vi "setting page.vi"(5 "NAN error":i32, 11 "error constant":errorcluster) -> (3 "sensor cluster":T5={"ch sensor1"=2.0, "ch sensor2"=3.0, "chs ensor3"=4.0, "ch sw sensor1"=0.0, "ch sw sensor2"=1.0}, 4 "This VI":refnum<vi>, 6 "grtbar":T3={"level1 thr"=5.0, "level2 thr"=10.0, "gr.th1"=900.0, "gr.th2"=900.0, "gr.th3"=900.0, "gr.th4"=900.0, "gr.th5"=18000.0, "gr.th6"=20000.0, "gr.th7"=21000.0, "gr.th8"=22000.0, "gr.th9"=3000.0, "def size"=5.0, "Frame False Thr"=280.0}, 8 "curv cluster":T2={"Thr1"=40000.0, "Thr2"=40000.0, "Thr3"=40000.0, "Port"=502.0, "time out"=50.0, "SWR thr"=20000.0, "SWL thr "=20000.0, "Curv thr (mm)"=13.0, "SW timout(s)"=0.25, "falling level thr"=59000.0, "denoise thr1"=20000.0, "denoise thr2"=20000.0, "denoise thr3"=20000.0, "low level read thr"=39000.0, "Debounce Time"=0.5}, 10 "IP # 2":string="169.254.116.245", 13 "general setting":T1={"plt number dis"=45, "Table Name"="pallet", "Database Name"="PALLETCAR", "DB days to save"=3}, 14 "counting role":T4(ring), 15 "img path 2":path=path "C:/Users/user/Pictures/saved pic")   [LabVIEW 2019]
panel:
  out "NAN Error":i32
  out "error constant 2":errorcluster
  out "Errors":string
  in  "DB days to save":i16=3
  in  "Debounce Time":dbl=0.5
  in  "counting role 2":T4(ring) caption="counting role"
  in  "Frame False Thr":dbl=280.0
  in  "ch sw sensor1":dbl
  out "Side Wall Setting":string
  in  "Port":dbl=502.0
  in  "SWL thr":dbl=20000.0
  in  "denoise thr3":dbl=20000.0
  in  "denoise thr2":dbl=20000.0
  in  "low level read thr":dbl=39000.0
  in  "denoise thr1":dbl=20000.0
  in  "falling level thr":dbl=59000.0
  in  "Database Name":string="PALLETCAR"
  in  "plt number dis":i16=45
  in  "Table Name":string="pallet"
  out "General Setting":string
  in  "SW timout(s)":dbl=0.25
  in  "Curv thr (mm)":dbl=13.0
  in  "SWR thr":dbl=20000.0
  in  "ch sw sensor2":dbl=1.0
  in  "chs ensor3":dbl=4.0
  in  "ch sensor2":dbl=3.0
  in  "ch sensor1":dbl=2.0
  in  "gr.th7":dbl=21000.0
  in  "gr.th8":dbl=22000.0
  in  "gr.th9":dbl=3000.0
  in  "Thr3":dbl=40000.0
  out "Gratebar Setting":string
  in  "gr.th6":dbl=20000.0
  in  "gr.th5":dbl=18000.0
  in  "gr.th4":dbl=900.0
  in  "gr.th3":dbl=900.0
  in  "gr.th2":dbl=870.0
  in  "gr.th1":dbl=850.0
  in  "IP #":string="169.254.116.245"
  out "Curve Setting":string
  in  "def size":dbl=5.0
  in  "Img Path":path=path "C:/Users/user/Pictures/saved pic"
  in  "level2 thr":dbl=50.0
  in  "level1 thr":dbl=25.0
  in  "time out":dbl=50.0
  in  "Thr2":dbl=40000.0
  in  "Thr1":dbl=40000.0
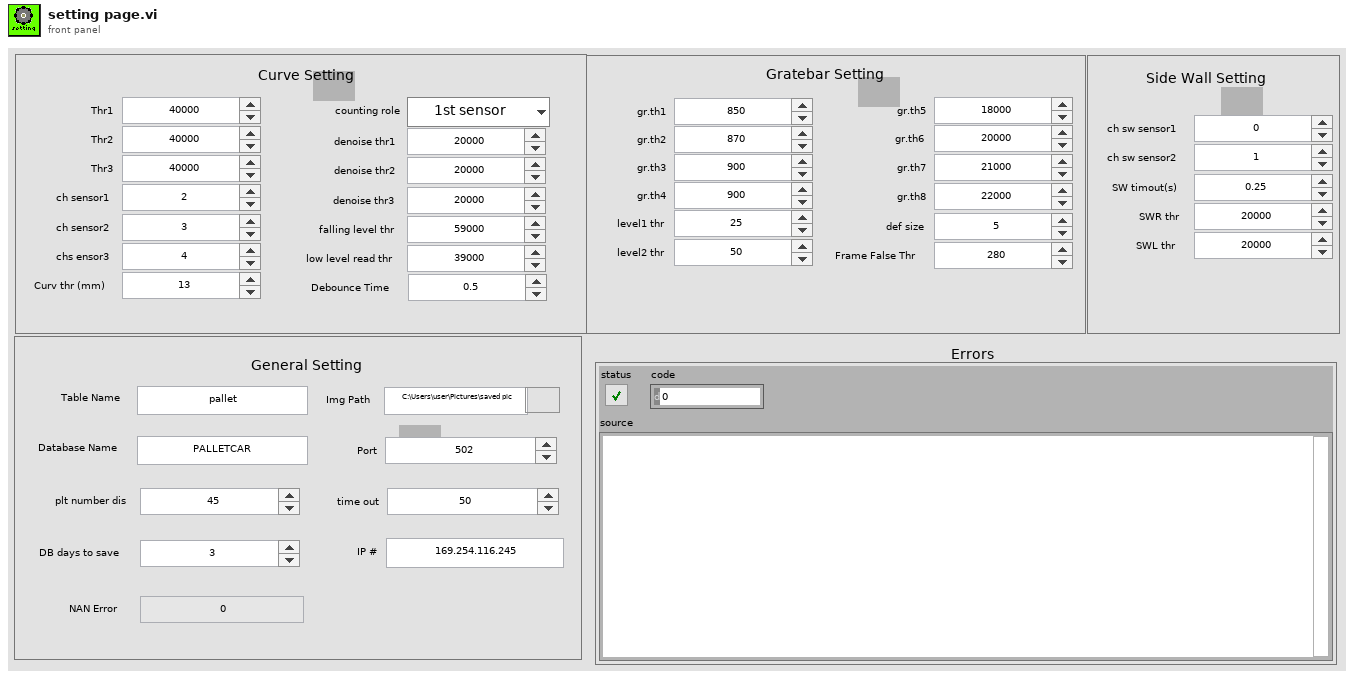
[diagram p1: front panel]
types:
  T1 = cluster{"plt number dis":i16, "Table Name":string, "Database Name":string, "DB days to save":i16}
  T2 = cluster{"Thr1":dbl, "Thr2":dbl, "Thr3":dbl, "Port":dbl, "time out":dbl, "SWR thr":dbl, "SWL thr ":dbl, "Curv thr (mm)":dbl, "SW timout(s)":dbl, "falling level thr":dbl, "denoise thr1":dbl, "denoise thr2":dbl, "denoise thr3":dbl, "low level read thr":dbl, "Debounce Time":dbl}
  T3 = cluster{"level1 thr":dbl, "level2 thr":dbl, "gr.th1":dbl, "gr.th2":dbl, "gr.th3":dbl, "gr.th4":dbl, "gr.th5":dbl, "gr.th6":dbl, "gr.th7":dbl, "gr.th8":dbl, "gr.th9":dbl, "def size":dbl, "Frame False Thr":dbl}
  T4 = enum16{"1st sensor", "2nd sensor", "3rd sensor", "1st+2nd", "1st+3rd", "2nd+3rd", "1st+2nd+3rd"}
  T5 = cluster{"ch sensor1":dbl, "ch sensor2":dbl, "chs ensor3":dbl, "ch sw sensor1":dbl, "ch sw sensor2":dbl}
  T6 = cluster{"plt number dis":i16, "Table Name":string}
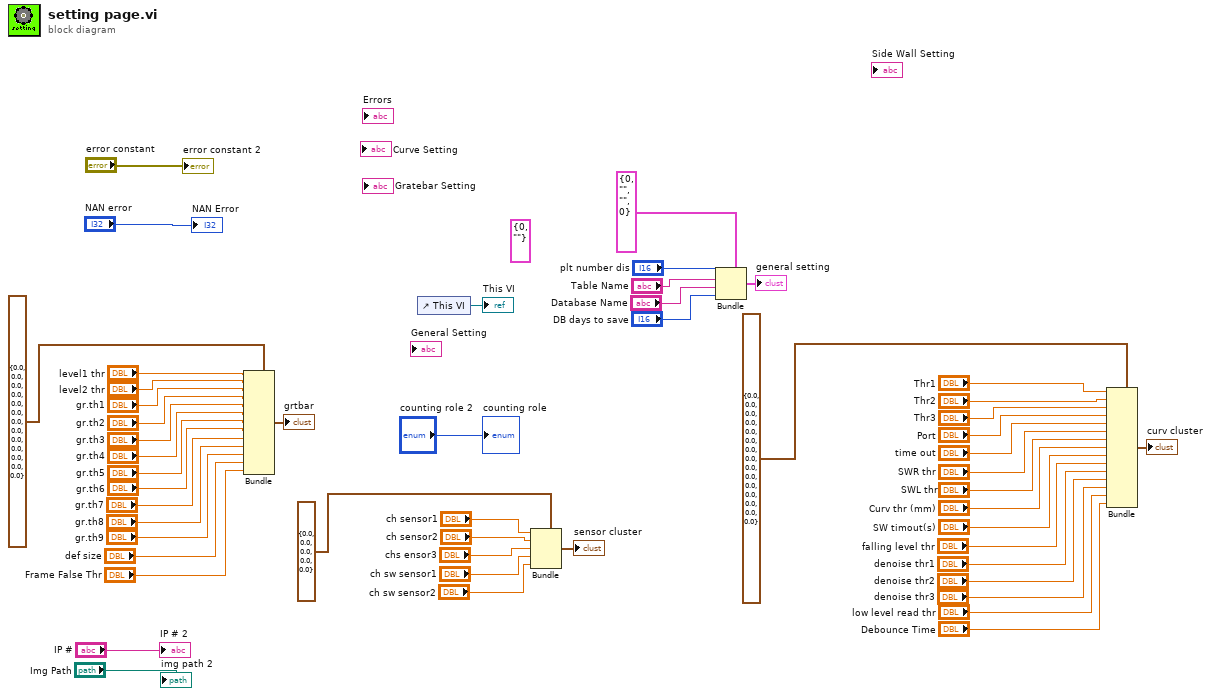
[diagram p0: block diagram]
diagram:
  (unwired) T6 {"plt number dis"=0, "Table Name"=""} ("cluster")
  n1 = Bundle(cluster=T3 {"level1 thr"=0.0, "level2 thr"=0.0, "gr.th1"=0.0, "gr.th2"=0.0, "gr.th3"=0.0, "gr.th4"=0.0, "gr.th5"=0.0, "gr.th6"=0.0, "gr.th7"=0.0, "gr.th8"=0.0, "gr.th9"=0.0, "def size"=0.0, "Frame False Thr"=0.0}, "level1 thr"="level1 thr", "level2 thr"="level2 thr", "gr.th1"="gr.th1", "gr.th2"="gr.th2", "gr.th3"="gr.th3", "gr.th4"="gr.th4", "gr.th5"="gr.th5", "gr.th6"="gr.th6", "gr.th7"="gr.th7", "gr.th8"="gr.th8", "gr.th9"="gr.th9", "def size"="def size", "Frame False Thr"="Frame False Thr") -> (→"grtbar":T3)
  n2 = control-ref of="This VI"() -> (→"This VI":refnum<vi>)
  n3 = Bundle(cluster=T5 {"ch sensor1"=0.0, "ch sensor2"=0.0, "chs ensor3"=0.0, "ch sw sensor1"=0.0, "ch sw sensor2"=0.0}, "ch sensor1"="ch sensor1", "ch sensor2"="ch sensor2", "chs ensor3"="chs ensor3", "ch sw sensor1"="ch sw sensor1", "ch sw sensor2"="ch sw sensor2") -> (→"sensor cluster":T5)
  n4 = Bundle(cluster=T1 {"plt number dis"=0, "Table Name"="", "Database Name"="", "DB days to save"=0}, "plt number dis"="plt number dis", "Table Name"="Table Name", "Database Name"="Database Name", "DB days to save"="DB days to save") -> (→"general setting":T1)
  n5 = Bundle(cluster=T2 {"Thr1"=0.0, "Thr2"=0.0, "Thr3"=0.0, "Port"=0.0, "time out"=0.0, "SWR thr"=0.0, "SWL thr "=0.0, "Curv thr (mm)"=0.0, "SW timout(s)"=0.0, "falling level thr"=0.0, "denoise thr1"=0.0, "denoise thr2"=0.0, "denoise thr3"=0.0, "low level read thr"=0.0, "Debounce Time"=0.0}, "Thr1"="Thr1", "Thr2"="Thr2", "Thr3"="Thr3", "Port"="Port", "time out"="time out", "SWR thr"="SWR thr", "SWL thr"="SWL thr", "Curv thr (mm)"="Curv thr (mm)", "SW timout(s)"="SW timout(s)", "falling level thr"="falling level thr", "denoise thr1"="denoise thr1", "denoise thr2"="denoise thr2", "denoise thr3"="denoise thr3", "low level read thr"="low level read thr", "Debounce Time"="Debounce Time") -> (→"curv cluster":T2)
  "IP # 2" <- "IP #"
  "img path 2" <- "Img Path"
  "counting role" <- "counting role 2"
  "error constant 2" <- "error constant"
  "NAN Error" <- "NAN error"
